vi "AudioTest.Graph, Compare Data Plots to Limit Plots.vi"(9 "Limit Names":string[](array[string]), 10 "Limits":cluster{"X":dbl[], "Y":dbl[]}[](array[cluster]), 11 "Data":cluster{"X":dbl[], "Y":dbl[]}[](array[cluster])) -> (3 "FAIL":bool)   [LabVIEW 2018]
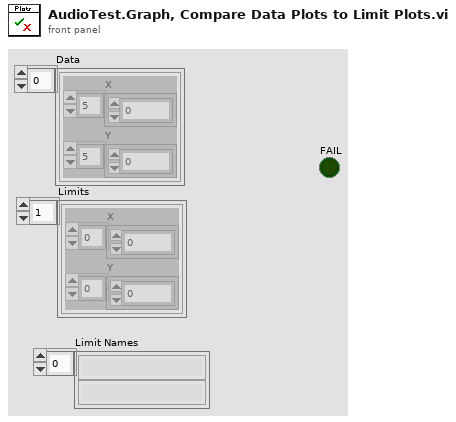
[diagram p1: front panel]
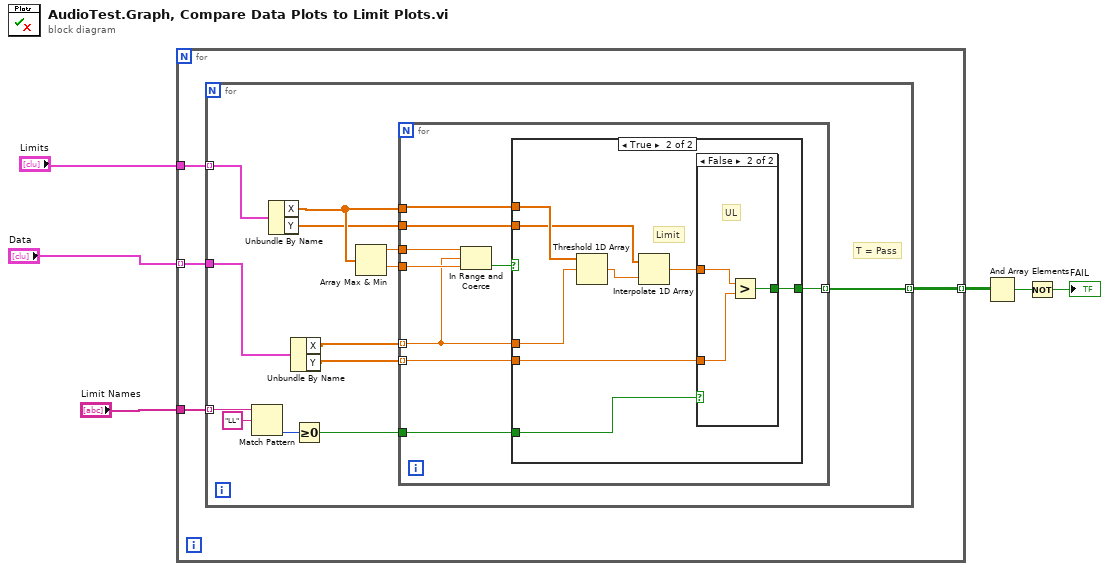
[diagram p0: block diagram]
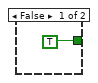
[diagram p2: hidden frame]
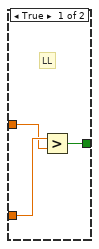
[diagram p3: hidden frame]
diagram:
  n1 = for {
    tunnel: "Data" -> [w10] mode=indexing
    tunnel: "Limits" -> [w9]
    tunnel: "Limit Names" -> [w8]
    tunnel: [w7] -> w1 mode=indexing
    n2 = for {
      tunnel: w10 -> [w17]
      tunnel: w9 -> [w14] mode=indexing
      tunnel: w8 -> [w21] mode=indexing
      tunnel: [w11] -> w7 mode=indexing
      # "T = Pass"
      n3 = Match Pattern(string=w21, regular expression="LL") -> (offset past match=w19:i32)  [unwired: 1 in, 3 out]
      n4 = Unbundle By Name(w14) -> ("X"=w13:dbl[], "Y"=w12:dbl[])
      n5 = Unbundle By Name(w17) -> ("X"=w16:dbl[], "Y"=w15:dbl[])
      n6 = Greater Or Equal To 0?(x=w19) -> (x >= 0?=w18:bool)
      n7 = Array Max & Min(array=w13) -> (max value=w23:dbl, min value=w22:dbl)  [unwired: 2 out]
      n8 = for {
        tunnel: w13 -> [w27]
        tunnel: w12 -> [w26]
        tunnel: w16 -> [w28] mode=indexing
        tunnel: w15 -> [w30] mode=indexing
        tunnel: w23 -> [w32]
        tunnel: w22 -> [w31]
        tunnel: [w25] -> w11 mode=indexing
        tunnel: w18 -> [w24]
        n9 = In Range and Coerce(upper limit=w32, x=w28, lower limit=w31) -> (In Range?=w29:bool)  [unwired: 1 out]
        n10 = case shown="True" w29 {
          tunnel: w30 -> [_ w37]
          tunnel: w28 -> [_ w40]
          tunnel: w27 -> [_ w41]
          tunnel: w26 -> [_ w38]
          tunnel: [TRUE w36] -> w25
          tunnel: w24 -> [_ w34]
          frame False {
          }
          frame True {
            # "Limit"
            n11 = Threshold 1D Array(2:w40, 3:w41) -> (0:w39:dbl)  [unwired: 1 in]
            n12 = Interpolate 1D Array(1:w39, 2:w38) -> (0:w35:dbl)
            n13 = case shown="False" w34 {
              tunnel: w35 -> [w43 w46]
              tunnel: w37 -> [w44 w45]
              tunnel: [w42 w47] -> w36
              frame True {
                # "LL"
                n14 = Greater?(x=w44, y=w43) -> (0:w42:bool)
              }
              frame False {
                # "UL"
                n15 = Greater?(x=w46, y=w45) -> (0:w47:bool)
              }
            }
          }
        }
      }
    }
  }
  n16 = And Array Elements(Boolean array=w1) -> (logical AND=w5:bool)
  n17 = Not(x=w5) -> (.not. x?=→"FAIL":bool)
